vi "Main_ttr.vi"() -> ()   [LabVIEW 2014]
uses:
  C:/Users/Avogadro/Desktop/VersaUSB/VersaUSB.dll
  VersaUSB.dll
panel:
  out "Error Message:":string
  out "VersaLase Reply":string
  in  "VersaLase Command/ Query":string
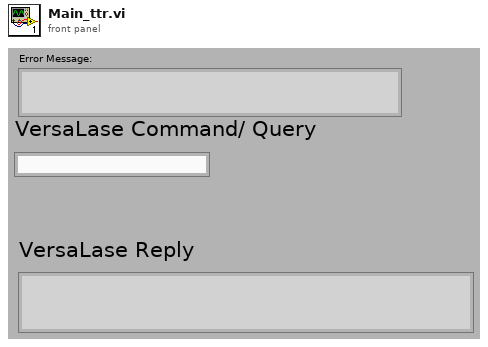
[diagram p1: front panel]
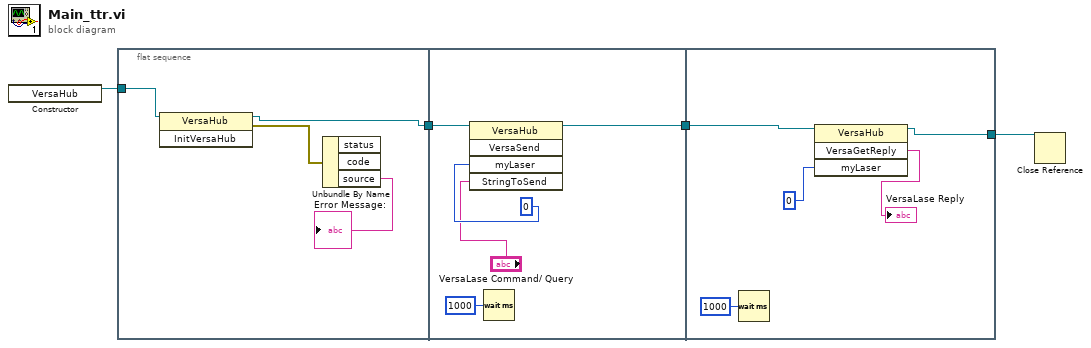
[diagram p0: block diagram]
diagram:
  n1 = constructor class="VersaHub"() -> (reference out=w4:refnum<k24>)  [unwired: 3 in, 2 out]
  n2 = flat-sequence {
    tunnel: w4 -> [w6]
    tunnel: [w5] -> w1
    tunnel: w1 -> [w11]
    tunnel: [w10] -> w2
    tunnel: [w16] -> w3
    tunnel: w2 -> [w15]
    frame #0 {
      n3 = invoke class="VersaHub" method="InitVersaHub"(reference=w6) -> (reference out=w5:refnum<k24>, error out=w8:errorcluster)  [unwired: 2 in, 1 out]
      n4 = Unbundle By Name(w8) -> ("source"=→"Error Message:":string)  [unwired: 2 out]
    }
    frame #1 {
      n5 = invoke class="VersaHub" method="VersaSend"(reference=w11, "myLaser"=0, "StringToSend"="VersaLase Command/ Query") -> (reference out=w10:refnum<k24>)  [unwired: 2 in, 4 out]
      n6 = Wait (ms)(milliseconds to wait=1000) -> ()  [unwired: 1 out]
    }
    frame #2 {
      n7 = Wait (ms)(milliseconds to wait=1000) -> ()  [unwired: 1 out]
      n8 = invoke class="VersaHub" method="VersaGetReply"(reference=w15, "myLaser"=0) -> (reference out=w16:refnum<k24>, "VersaGetReply"=→"VersaLase Reply":string)  [unwired: 2 in, 2 out]
    }
  }
  n9 = Close Reference(reference=w3) -> ()  [unwired: 1 in, 1 out]
